vi "LEIN Arbeiter.vi"(1 "LEIN m Serial Transmitt Loop ID":i32, 11 "error Inn":errorcluster) -> ()   [LabVIEW 2011]
uses:
  Defenitions/LEIN cycle holder.ctl
  Defenitions/LEIN CMD Cluster.ctl
  Defenitions/LEIN CMD List.ctl
  Defenitions/LEIN Reply Holder.ctl
  Defenitions/LEIN custom reply Q.ctl
  GUI/Options/Modem simulation setup.ctl
  Measurments Handling/Common/Variable List Common Digital.ctl
  Measurments Handling/Action Analog Handler.ctl
  emi Lib/Basic/0 - General/Error/Private/_emi_Filter type.ctl
  <vilib>/Instr/_visa.llb/VISA Flush IO Buffer Mask.ctl
  emi Lib/Basic/0 - General/Error/Private/emi_Error Filter Single.vi
  emi Lib/System 01/0 - General/App/Loop control 2/Private/_emi_ SMLoop start condition.vi
  emi Lib/System 01/0 - General/App/Loop control 2/Private/_emi_ SMLoop Error Check.vi
  emi Lib/System 01/0 - General/App/Loop control 2/Private/_emi_SMLoop Register new.vi
  emi Lib/System 01/0 - General/S&E reporting/emi_Send S&E Error message.vi
  emi Lib/Basic/0 - General/Error/emi_ Is Error state.vi
  emi Lib/System 01/0 - General/emi_Read System ID.vi
  emi Lib/System 01/0 - General/App/Loop control/Private/_emi_GFV Loop Linking.vi
  emi Lib/System 01/0 - General/App/Loop control/Private/_emi_GFV Loop Enable.vi
  emi Lib/System 01/0 - General/App/Loop control 2/Private/_emi_ SMLoop Restart.vi
  emi Lib/System 01/0 - General/App/Private/_emi_GFV App Close.vi
  emi Lib/System 01/0 - General/App/Loop control 2/Private/_emi_ SMLoop Restart Counter.vi
  emi Lib/System 01/0 - General/App/Loop control/Private/_emi_GFV Loop Running.vi
  emi Lib/System 01/0 - General/Private/_emi_GFV System ID.vi
  emi Lib/System 01/0 - General/S&E reporting/Private/_emi_S&E Q Generator.vi
  emi Lib/System 01/0 - General/App/Loop control/Private/_emi_GFV stop a loop so it can reset.vi
panel:
  out "Numb sent":i32 format="%.0x"
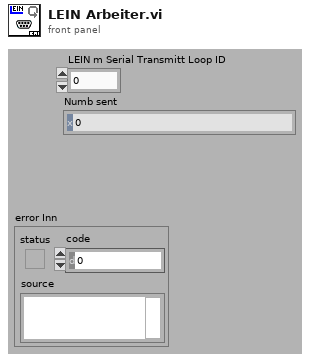
[diagram p1: front panel]
types:
  T1 = typedef "LEIN cycle holder.ctl" = cluster{"CMD":T2, "Retry if  unsucessful":bool, "LEIN reply holder":T4, "Reply in custom Q":bool, "LEIN custom reply Q":T5}
  T2 = typedef "LEIN CMD Cluster.ctl" = cluster{"SID":u8, "ANF":bool, "CMD":T3, "DATA":u8[]}
  T3 = typedef "LEIN CMD List.ctl" = enum8{"ACTI", "TASK", "RES0", "STAT", "RES1", "RES2", "RES3", "USER"}
  T4 = typedef "LEIN Reply Holder.ctl" = cluster{"Reply msg(cmdif no reply)":T2, "Reply time":timestamp, "Valid reply":bool}
  T5 = typedef "LEIN custom reply Q.ctl" = refnum<queue>
  T6 = typedef "Variable List Common Digital.ctl" = enum16{"PCP Connected", "PCP PC Control", "HV PSU connected", "HV PSU HV Active", "Modem Connected", "Tool Connected", "CanBus interface"}
  T7 = typedef "Action Analog Handler.ctl" = enum16{"GET value", "GET Single Frequenzy", "GET All Values", "GET Waveform", "Get Numb Var", "SET Value", "START Buffer", "REG Variable", "BUF size(total antal sekund)", "PULS", "Get a Value at time", "Set initial waveform"}
  T8 = typedef "_emi_Filter type.ctl" = enum16{"Error&Warning", "Warning", "Error"}
  T9 = typedef "_emi_ SMLoop sates.ctl" = enum16{"Init", "Standby", "Start", "Normal Operation", "Stop", "Error Handling", "End", "Post"}
  T10 = typedef "Modem simulation setup.ctl" = cluster{"Modem dealay sim":bool, "Sim baud Tx":u16, "Bit Error fraction Tx":dbl, "Sim baud Rx":u16, "Bit Error fraction Rx":dbl}
  T11 = cluster{"VISA name":refnum<visa-resource-name>, "Modem sim":T10}
  T12 = typedef "Status Digitalish.ctl" = enum16{"NA", "False", "True"}
  T13 = typedef "VISA Flush IO Buffer Mask.ctl" = u16
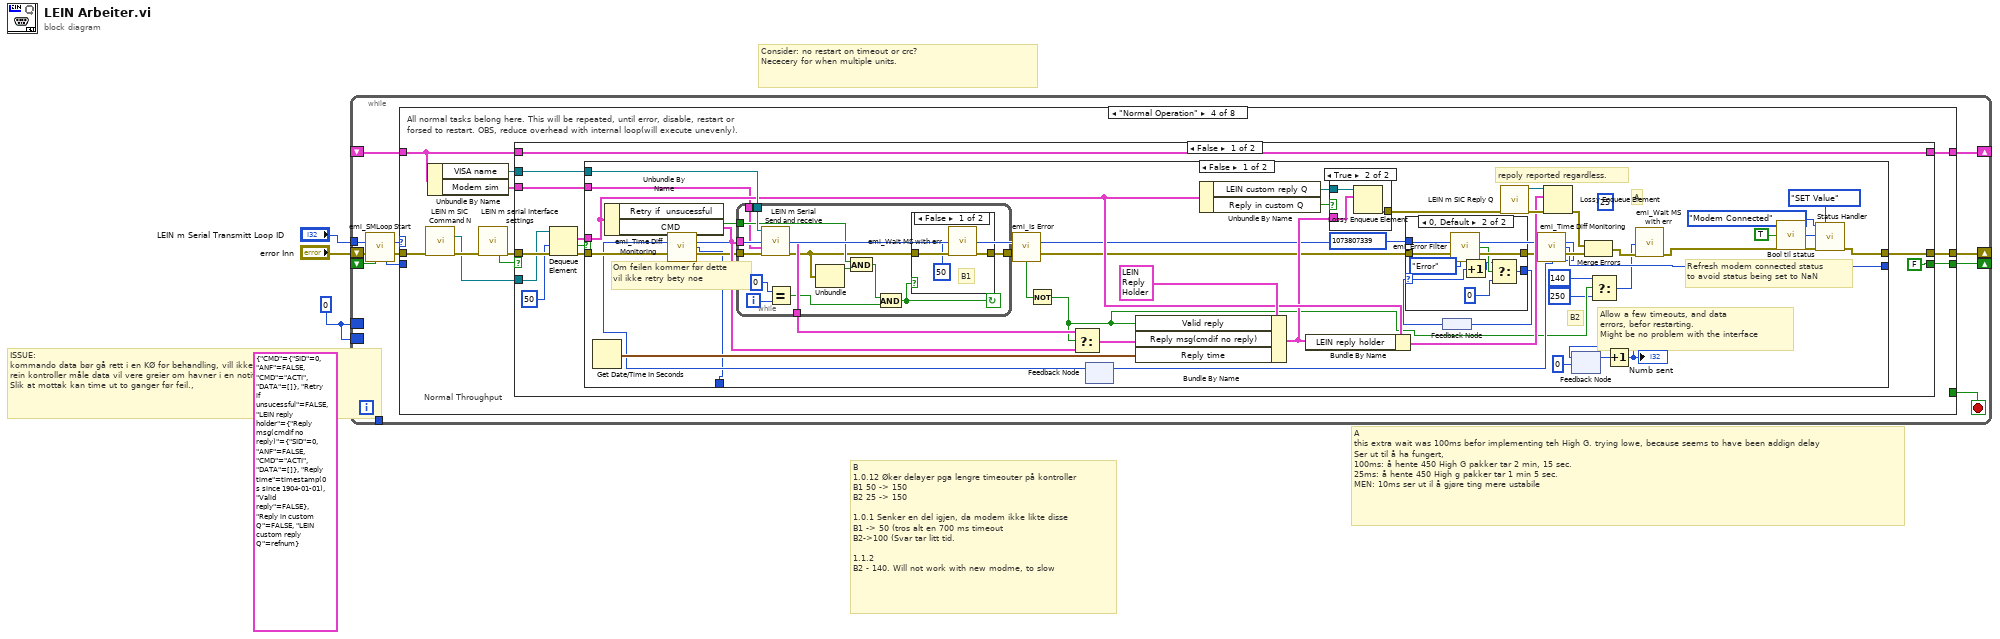
[diagram p0: block diagram]
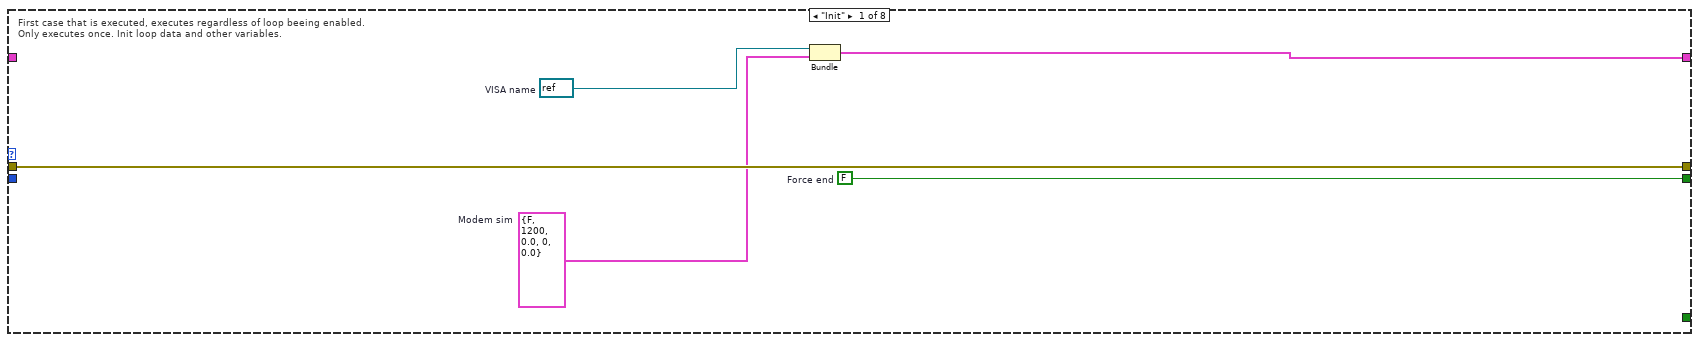
[diagram p2: hidden frame]
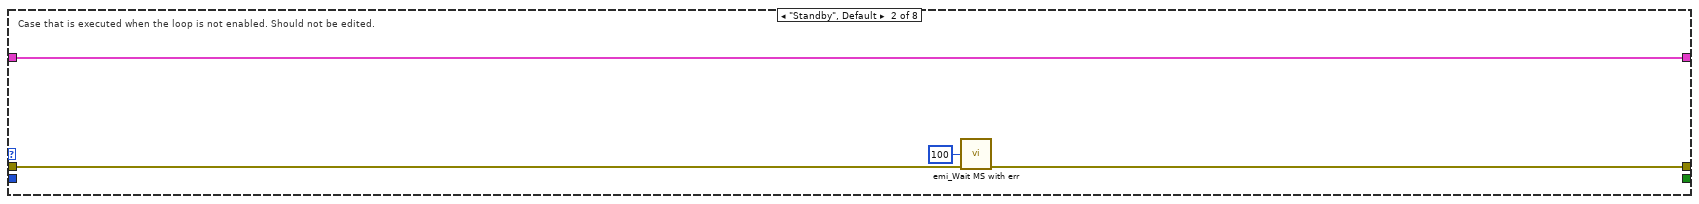
[diagram p3: hidden frame]
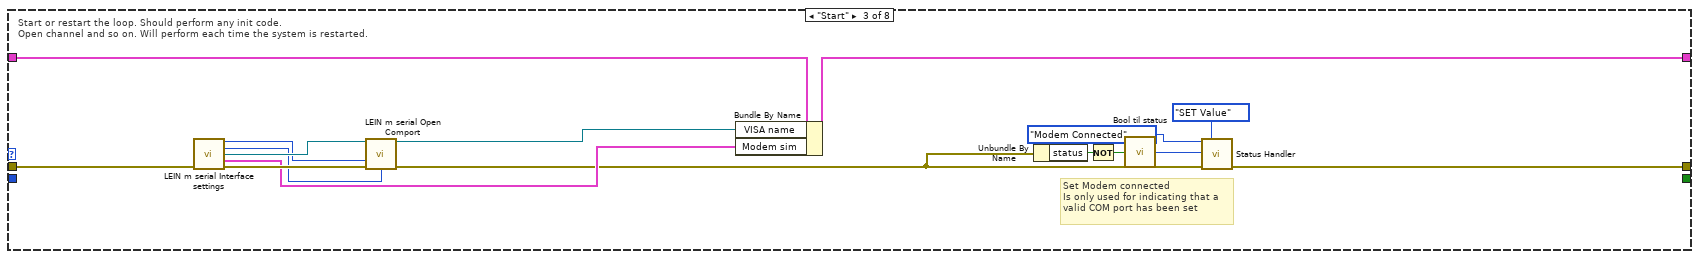
[diagram p4: hidden frame]
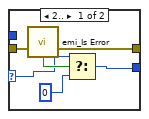
[diagram p5: hidden frame]
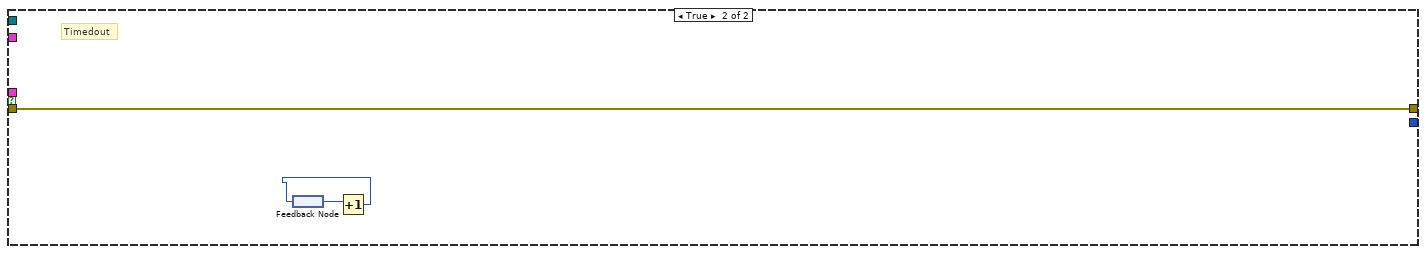
[diagram p8: hidden frame]
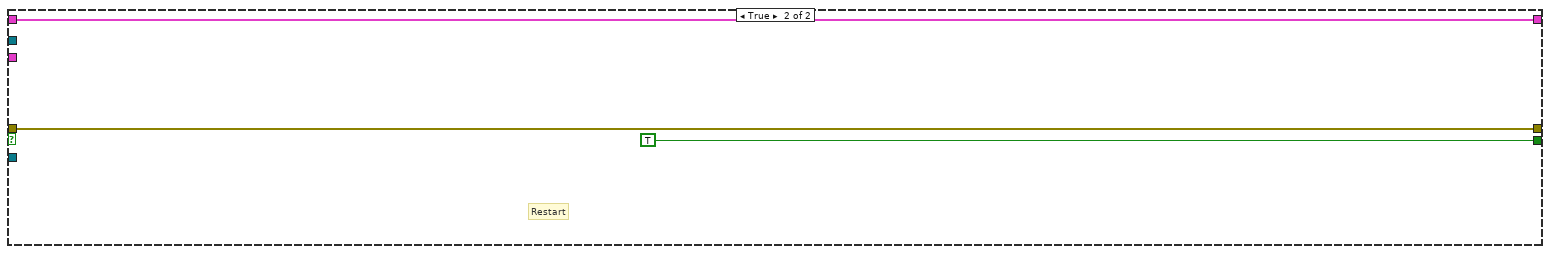
[diagram p9: hidden frame]
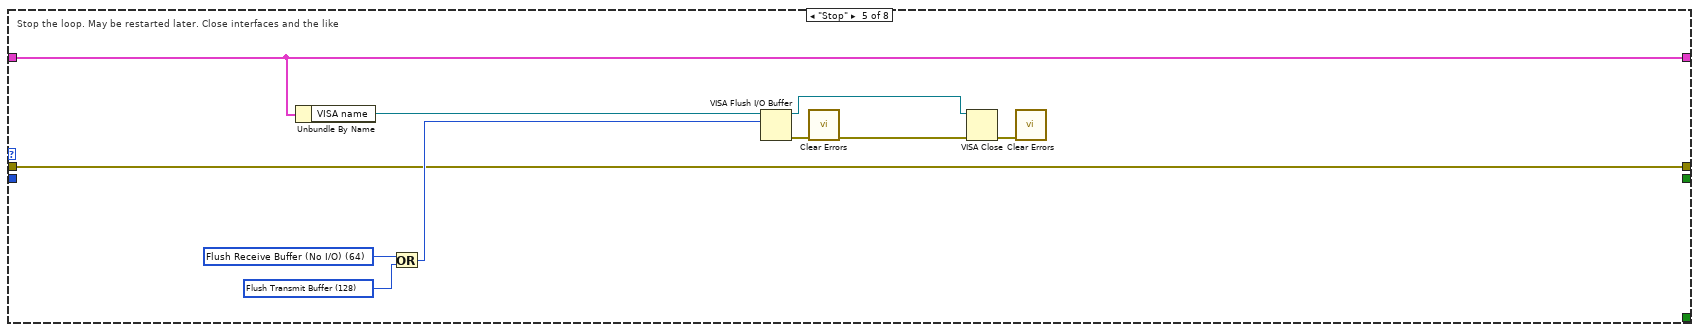
[diagram p10: hidden frame]
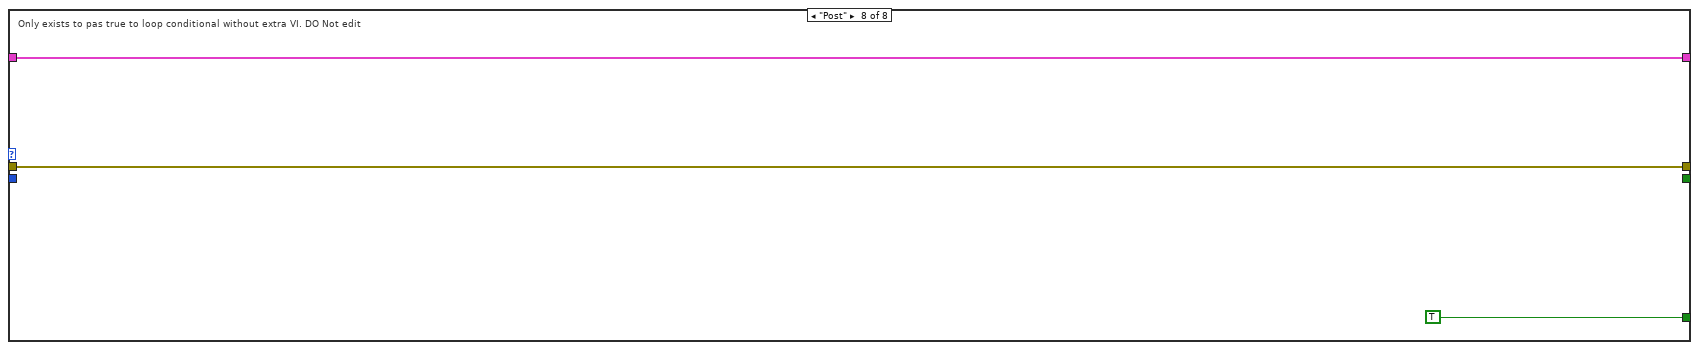
[diagram p13: hidden frame]
diagram:
  w1 = 0
  (unwired) T1 {"CMD"={"SID"=0, "ANF"=FALSE, "CMD"=enum."ACTI", "DATA"=[]}, "Retry if  unsucessful"=FALSE, "LEIN reply holder"={"Reply msg(cmdif no reply)"={"SID"=0, "ANF"=FALSE, "CMD"=enum."ACTI", "DATA"=[]}, "Reply time"=timestamp(0 s since 1904-01-01), "Valid reply"=FALSE}, "Reply in custom Q"=FALSE, "LEIN custom reply Q"=refnum} ("element")
  # "B\n1.0.12 Øker delayer pga lengre timeouter på kontroller\nB1 50 -> 150\nB2 25 -> 150\n\n1.0.1 Senker en del igjen, da modem ikke likte disse\nB1 -> 50 (tros alt en 700 ms timeout\nB2->100 (Svar tar litt tid.\n\n1.1.2\nB2 - 140. Will not work with new modme, to slow"
  # "A \nthis extra wait was 100ms befor implementing teh High G. trying lowe, because seems to have been addign delay\nSer ut til å ha fungert,  \n100ms: å hente 450 High G pakker tar 2 min, 15 sec.\n25ms: å hente 450 High g pakker tar 1 min 5 sec.\nMEN: 10ms ser ut il å gjøre ting mere ustabile"
  # "Consider: no restart on timeout or crc?\nNececery for when multiple units."
  # "ISSUE:\nkommando data bør gå rett i en KØ for behandling, vill ikke gå glipp av noe,\nrein kontroller måle data vil vere greier om havner i en notifier.\nSlik at mottak kan time ut to ganger før feil.,"
  n1 = while {
    shift-right: [w15] -> _
    shift-left: _ -> [w11]
    shift-right: [w13] -> _
    shift-left: "error Inn" -> [w9]
    tunnel: [w12] -> _
    shift-right: [w10] -> _
    shift-left: _ -> [w6]
    tunnel: "LEIN m Serial Transmitt Loop ID" -> [w7]
    border: w1 -> [_]
    border: w1 -> [_]
    i -> [w12]
    stop <- w14 stop-if-true
    n2 = call "emi_SMLoop Start.vi"("Loop ID"=w7, "error in (no error)"=w9, "Force Stop(F)"=w6) -> ("Loop command"=w4:T9, "error out"=w8:errorcluster, "Loop ID out"=w5:i32)  [unwired: 10 in]
    n3 = case shown="\"Normal Operation\"" w4 {
      tunnel: [w19 w21 w39 w49 w151 w162 w163 w166] -> w15
      tunnel: [_ _ _ _ _ _ _ TRUE] -> w14
      tunnel: w8 -> [w20 w23 w38 w51 w152 w161 w164 w167]
      tunnel: [w20 w22 w26 w50 w152 w161 w164 w167] -> w13
      tunnel: w11 -> [_ w21 w40 w48 w151 w162 w163 w166]
      tunnel: [w18 _ _ w47 _ _ _ _] -> w10
      tunnel: w5 -> [_ _ _ _ _ _ _ _]
      frame "Init" {
        w16 = T10 {"Modem dealay sim"=FALSE, "Sim baud Tx"=1200, "Bit Error fraction Tx"=0.0, "Sim baud Rx"=0, "Bit Error fraction Rx"=0.0}  # Modem sim
        w17 = refnum<visa-resource-name> refnum  # VISA name
        w18 = FALSE  # Force end
        # "First case that is executed, executes regardless of loop beeing enabled.\nOnly executes once. Init loop data and other variables."
        n4 = Bundle("VISA name"=w17, "Modem sim"=w16) -> (w19:T11)  [unwired: 1 in]
      }
      frame "Standby", Default {
        # "Case that is executed when the loop is not enabled. Should not be edited."
        n5 = call "emi_Wait MS with err.vi"("milliseconds to wait(0)"=u32 100, "error in (no error)"=w23) -> ("error out"=w22:errorcluster)  [unwired: 13 in]
      }
      frame "Start" {
        # "Set Modem connected\nIs only used for indicating that a\nvalid COM port has been set"
        # "Start or restart the loop. Should perform any init code. \nOpen channel and so on. Will perform each time the system is restarted."
        n6 = call "LEIN m serial Interface settings.vi"("error in (no error)"=w38) -> ("baud rate out"=w34:u32, "Timeout out"=w33:u32, "LEIN m  Visa name  out"=w36:refnum<visa-resource-name>, "Modem sim out"=w32:T10, "error out"=w37:errorcluster)  [unwired: 9 in, 1 out]
        n7 = call "LEIN m serial Open Comport.vi"("Comport"=w36, "baud rate (9600)"=w34, "error in (no error)"=w37, "Reply timeout (1000 ms)"=w33) -> ("VISA resource name out"=w35:refnum<visa-resource-name>, "error out"=w25:errorcluster)  [unwired: 10 in]
        n8 = Bundle By Name(cluster=w40, "VISA name"=w35, "Modem sim"=w32) -> (w39:T11)
        n9 = Unbundle By Name(w25) -> ("status"=w28:bool)
        n10 = Not(x=w28) -> (.not. x?=w27:bool)
        n11 = call "Bool til status.vi"("Boolean"=w27) -> ("Status"=w29:T12)  [unwired: 8 in]
        n12 = call "Status Handler.vi"("Variable Index"=Variable_List_Common_Digital."Modem Connected" ("Action"), "Action"=Action_Analog_Handler."SET Value" ("Action(GET)"), "Value"=w29, "error in (no error)"=w25) -> ("error out"=w26:errorcluster)  [unwired: 7 in, 4 out]
      }
      frame "Normal Operation" {
        # "Normal Throughput"
        # "All normal tasks belong here. This will be repeated, until error, disable, restart or\nforsed to restart. OBS, reduce overhead with internal loop(will execute unevenly)."
        n13 = call "LEIN m SIC Command N.vi"("error in (no error)"=w51) -> ("queue out"=w43:refnum<queue>, "error out"=w45:errorcluster)  [unwired: 13 in]
        n14 = Unbundle By Name(w48) -> ("VISA name"=w44:refnum<visa-resource-name>, "Modem sim"=w41:T10)
        n15 = call "LEIN m serial Interface settings.vi"("error in (no error)"=w45) -> ("Changed since last get"=w42:bool, "error out"=w46:errorcluster)  [unwired: 9 in, 4 out]
        n16 = case shown="False" w42 {
          tunnel: [FALSE ("Force End") TRUE ("Force End")] -> w47
          tunnel: [w54 w149] -> w50
          tunnel: w46 -> [w60 w149]
          tunnel: [w61 w148] -> w49
          tunnel: w48 -> [w61 w148]
          tunnel: w44 -> [w56 _]
          tunnel: w43 -> [w55 _]
          tunnel: w41 -> [w52 _]
          frame False {
            n17 = Dequeue Element(queue=w55, timeout in ms (-1)=50, error in (no error)=w60) -> (element=w57:T1, timed out?=w58:bool, error out=w59:errorcluster)  [unwired: 1 out]
            n18 = case shown="False" w58 {
              tunnel: w59 -> [w108 w147]
              tunnel: [w63 w147] -> w54
              tunnel: w57 -> [w93 _]
              tunnel: w56 -> [w107 _]
              tunnel: w52 -> [w81 _]
              tunnel: [w75 _] -> _
              tunnel: [w74 _] -> _
              frame False {
                (unwired) u32 25 ("millisecond multiple(0)")
                # "Refresh modem connected status\nto avoid status being set to NaN"
                # "B2"
                # "A"
                # "Allow a few timeouts, and data \nerrors, befor restarting.\nMight be no problem with the interface"
                # "Om feilen kommer før dette\nvil ikke retry bety noe"
                # "repoly reported regardless."
                n19 = Get Date/Time In Seconds() -> (seconds since 1Jan1904=w104:timestamp)
                n20 = Unbundle By Name(w93) -> ("Retry if  unsucessful"=w99:bool, "CMD"=w84:T2)
                n21 = feedback #1() -> (w76:u32)  [unwired: 1 in]
                n22 = call "emi_Time Diff Monitoring.vi"("Previous Time"=w76, "error in (no error)"=w108) -> ("Current Time"=w77:u32, "Time Difference(ms)"=w75:u32, "error out"=w80:errorcluster)  [unwired: 11 in]
                n23 = while {
                  tunnel: w80 -> [w140]
                  tunnel: w107 -> [w139]
                  tunnel: [w128] -> w98
                  tunnel: [w138] -> w85
                  tunnel: w84 -> [w137]
                  tunnel: w99 -> [w132]
                  tunnel: w81 -> [w127]
                  i -> [w136]
                  stop <- w130 continue-if-true
                  n24 = call "LEIN m Serial Send and receive.vi"("VISA name"=w139, "CMD"=w137, "Modem sim(Off)"=w127, "error in"=w140) -> ("Reply"=w138:T2, "error out"=w129:errorcluster)  [unwired: 9 in, 1 out]
                  n25 = Equal?(x=0, y=w136) -> (x = y?=w134:bool)
                  n26 = Unbundle(w129) -> ("status"=w133:bool)  [unwired: 2 out]
                  n27 = And(x=w132, y=w133) -> (x .and. y?=w131:bool)
                  n28 = And(x=w131, y=w134) -> (x .and. y?=w130:bool)
                  n29 = case shown="False" w130 {
                    tunnel: w129 -> [w143 w144]
                    tunnel: [w142 w144] -> w128
                    frame False {
                      # "B1"
                      n30 = call "emi_Wait MS with err.vi"("milliseconds to wait(0)"=u32 50, "error in (no error)"=w143) -> ("error out"=w142:errorcluster)  [unwired: 13 in]
                    }
                    frame True {
                    }
                  }
                }
                n31 = call "emi_Is Error.vi"("error in (no error)"=w98) -> ("error out"=w89:errorcluster, "Is Error"=w97:bool)  [unwired: 13 in]
                n32 = Not(x=w97) -> (.not. x?=w72:bool)
                n33 = Select(t=w85, s=w72, f=w84) -> (s? t:f=w83:T2)
                n34 = Bundle By Name(cluster=T4 {"Reply msg(cmdif no reply)"={"SID"=0, "ANF"=FALSE, "CMD"=enum."ACTI", "DATA"=[]}, "Reply time"=timestamp(0 s since 1904-01-01), "Valid reply"=FALSE} ("LEIN reply holder"), "Valid reply"=w72, "Reply msg(cmdif no reply)"=w83, "Reply time"=w104) -> (w91:T4)
                n35 = Unbundle By Name(w93) -> ("LEIN custom reply Q"=w95:T5, "Reply in custom Q"=w96:bool)
                n36 = Bundle By Name(cluster=w93, "LEIN reply holder"=w91) -> (w92:T1)
                n37 = case shown="True" w96 {
                  tunnel: w95 -> [_ w126]
                  tunnel: w91 -> [_ w125]
                  tunnel: [_ w124] -> w90
                  frame False {
                  }
                  frame True {
                    n38 = Lossy Enqueue Element(queue=w126, element=w125) -> (error out=w124:errorcluster)  [unwired: 1 in, 3 out]
                  }
                }
                n39 = feedback #2() -> (w87:i32)
                n40 = case shown="0, Default" w87 {
                  selector: w87 -> [w110 w115]
                  tunnel: w89 -> [w114 w123]
                  tunnel: [w109 w122] -> w79
                  tunnel: 1073807339 ("Error Code") -> [_ w121]
                  tunnel: [w112 w117] -> w86
                  frame 2.. {
                    n41 = call "emi_Is Error.vi"("error in (no error)"=w114) -> ("error out"=w109:errorcluster, "Is Error"=w111:bool)  [unwired: 13 in]
                    n42 = Select(t=w110, s=w111, f=0) -> (s? t:f=w112:i32)
                  }
                  frame 0, Default {
                    n43 = call-poly "emi_Error Filter.vi"("Error Code"=w121, "error in (no error)"=w123, "Filter(Error&Warning)"=_emi_Filter_type."Error") -> ("Filter Triggered"=w119:bool, "error out"=w122:errorcluster)  [unwired: 11 in]
                    n44 = Increment(x=w115) -> (x+1=w118:i32)
                    n45 = Select(t=w118, s=w119, f=0) -> (s? t:f=w117:i32)
                  }
                }
                n46 = feedback-in #2(w86) -> ()
                n47 = call "LEIN m SIC Reply Q.vi"("error in (no error)"=w90) -> ("reply Q"=w105:refnum<queue>, "error out"=w106:errorcluster)  [unwired: 13 in]
                n48 = call "emi_Time Diff Monitoring.vi"("Previous Time"=w77, "error in (no error)"=w79) -> ("Current Time"=w73:u32, "Time Difference(ms)"=w74:u32, "error out"=w78:errorcluster)  [unwired: 11 in]
                n49 = feedback-in #1(w73) -> ()
                n50 = Lossy Enqueue Element(queue=w105, element=w92, error in (no error)=w106) -> (error out=w100:errorcluster)  [unwired: 3 out]
                n51 = feedback #3(0) -> (w101:i32)
                n52 = Merge Errors(w100, w78) -> (w82:errorcluster)
                n53 = Select(t=u32 140 ("millisecond multiple(0)"), s=w72, f=u32 250 ("millisecond multiple(0)")) -> (s? t:f=w69:u32)
                n54 = Increment(x=w101) -> (x+1=w102:i32)
                "Numb sent" <- w102
                n55 = feedback-in #3(w102) -> ()
                n56 = call "emi_Wait MS with err.vi"("milliseconds to wait(0)"=w69, "error in (no error)"=w82) -> ("error out"=w64:errorcluster)  [unwired: 13 in]
                n57 = call "Bool til status.vi"("Boolean"=TRUE) -> ("Status"=w65:T12)  [unwired: 8 in]
                n58 = call "Status Handler.vi"("Variable Index"=Variable_List_Common_Digital."Modem Connected" ("Action"), "Action"=Action_Analog_Handler."SET Value" ("Action(GET)"), "Value"=w65, "error in (no error)"=w64) -> ("error out"=w63:errorcluster)  [unwired: 7 in, 4 out]
              }
              frame True {
                # "Timedout"
                n59 = feedback #4() -> (w146:i32)
                n60 = Increment(x=w146) -> (x+1=w145:i32)
                n61 = feedback-in #4(w145) -> ()
              }
            }
          }
          frame True {
            # "Restart"
          }
        }
      }
      frame "Stop" {
        w153 = T13 128 items=["Flush Receive Buffer"=16, "Write Transmit Buffer to Device"=32, "Flush Receive Buffer (No I/O)"=64, "Flush Transmit Buffer"=128] ("Mask")
        w155 = T13 64 items=["Flush Receive Buffer"=16, "Write Transmit Buffer to Device"=32, "Flush Receive Buffer (No I/O)"=64, "Flush Transmit Buffer"=128] ("Mask")
        # "Stop the loop. May be restarted later. Close interfaces and the like"
        n62 = Unbundle By Name(w151) -> ("VISA name"=w157:refnum<visa-resource-name>)
        n63 = Or(x=w155, y=w153) -> (x .or. y?=w154:T13)
        n64 = VISA Flush I/O Buffer(VISA resource name=w157, mask (16)=w154) -> (VISA resource name out=w156:refnum<visa-resource-name>, error out=w158:errorcluster)  [unwired: 1 in]
        n65 = call <vilib>:"Clear Errors.vi"("error in (no error)"=w158) -> ("error out"=w159:errorcluster)  [unwired: 6 in]
        n66 = VISA Close(VISA resource name=w156, error in (no error)=w159) -> (error out=w160:errorcluster)
        n67 = call <vilib>:"Clear Errors.vi"("error in (no error)"=w160) -> ()  [unwired: 6 in, 1 out]
      }
      frame "Error Handling" {
        # "Loop automaticaly returns here after error is found. If error is cleared, \nLoop wil continue as normal(if was operative when error."
      }
      frame "End" {
        # "Only executes at application end has. Should performa any action the loop \nneeds to finnish. Executes only once."
      }
      frame "Post" {
        # "Only exists to pas true to loop conditional without extra VI. DO Not edit"
      }
    }
  }
